vi "CRYTS Step Move Up.vi"(11 "TreeRefereneIn":refnum<vi>) -> ()   [LabVIEW 2013]
panel:
  out "TreeRefereneOut":refnum<vi>
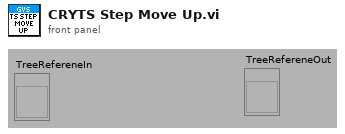
[diagram p1: front panel]
types:
  T1 = enum16{"Insert", "Remove", "Move up", "Move down"}
  T2 = cluster{"SourceRowNum":i32, "SourceCount":i32, "TargetRowNum":i32, "bResult":bool, "EditRowNum":i32}
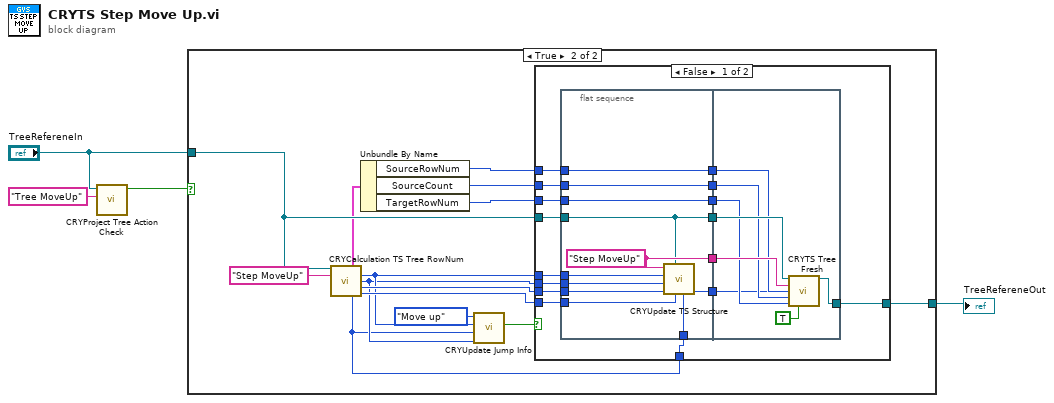
[diagram p0: block diagram]
diagram:
  n1 = call "CRYProject Tree Action Check.vi"("sOption"="Tree MoveUp", "Project Tree reference"="TreeRefereneIn") -> ("bResult"=w3:bool)  [unwired: 8 in, 1 out]
  n2 = case shown="True" w3 {
    tunnel: "TreeRefereneIn" -> [w5 w13]
    tunnel: [w5 w12] -> w1
    frame False {
    }
    frame True {
      n3 = call "CRYCalculation TS Tree RowNum.vi"("Tree Task SequenceIn"=w13, "sOption"="Step MoveUp") -> ("DispInfo Cluster Out"=w10:T2, "SourceRowNum"=w16:i32, "SourceCount"=w15:i32, "TargetRowNum"=w18:i32, "MoveCount"=w6:i32, "EditRowNum"=w17:i32)  [unwired: 7 in, 1 out]
      n4 = Unbundle By Name(w10) -> ("SourceRowNum"=w9:i32, "SourceCount"=w8:i32, "TargetRowNum"=w7:i32)
      n5 = call "CRYUpdate Jump Info.vi"("SourceCount"=w15, "MoveCount"=w6, "Step number Selected"=w16, "Action"=T1."Move up") -> ("Canceled?"=w11:bool)  [unwired: 6 in, 1 out]
      n6 = case shown="False" w11 {
        tunnel: w18 -> [w35 _]
        tunnel: w17 -> [w34 _]
        tunnel: w16 -> [w33 _]
        tunnel: w15 -> [w32 _]
        tunnel: w13 -> [w28 w54]
        tunnel: [w31 w54] -> w12
        tunnel: w9 -> [w26 _]
        tunnel: w8 -> [w24 _]
        tunnel: w7 -> [w22 _]
        tunnel: w6 -> [w20 _]
        frame False {
          n7 = flat-sequence {
            tunnel: [w44] -> w30
            tunnel: [w37] -> w29
            tunnel: [w41] -> w27
            tunnel: [w40] -> w25
            tunnel: [w39] -> w23
            tunnel: [w38] -> w21
            tunnel: w20 -> [w36]
            tunnel: w35 -> [w38]
            tunnel: w34 -> [w45]
            tunnel: w33 -> [w43]
            tunnel: w32 -> [w42]
            tunnel: w28 -> [w37]
            tunnel: w26 -> [w41]
            tunnel: w24 -> [w40]
            tunnel: w22 -> [w39]
            tunnel: w30 -> [w51]
            tunnel: w29 -> [w50]
            tunnel: w27 -> [w49]
            tunnel: w25 -> [w48]
            tunnel: w23 -> [w47]
            tunnel: w21 -> [w46]
            tunnel: [w52] -> w31
            frame #0 {
              w44 = "Step MoveUp" ("sOption")
              n8 = call "CRYUpdate TS Structure.vi"("Move Count"=w36, "Edit Step Num"=w45, "Tree Task SequenceIn"=w37, "Target Index"=w38, "Count"=w42, "Source Index"=w43, "sOption"=w44) -> ()  [unwired: 5 in]
            }
            frame #1 {
              n9 = call "CRYTS Tree Fresh.vi"("SequenceTree"=w50, "Edit Index"=w46, "sOption"=w51, "Source Index"=w49, "SourceCount"=w48, "Target Index"=w47, "Is Refresh?"=TRUE) -> ("SequenceTree out"=w52:refnum<vi>)  [unwired: 8 in]
            }
          }
        }
        frame True {
        }
      }
    }
  }
  "TreeRefereneOut" <- w1
